vi "测试-图片插入word.vi"() -> ()   [LabVIEW 2018]
uses:
  <vilib>/Utility/NIReport.llb/Report Type.ctl
  <vilib>/Utility/NIReport.llb/Append Image to Report (path wrap).vi
  <vilib>/Utility/NIReport.llb/NI_report.lvclass
  <vilib>/Utility/NIReport.llb/Word/NI_Word.lvclass
  <vilib>/Utility/NIReport.llb/NI_ReportGenerationCore.lvlib
panel:
  out "报告生成路径 2":path
  out "报告生成路径":path
  out "标注图":T1(plugin-control)
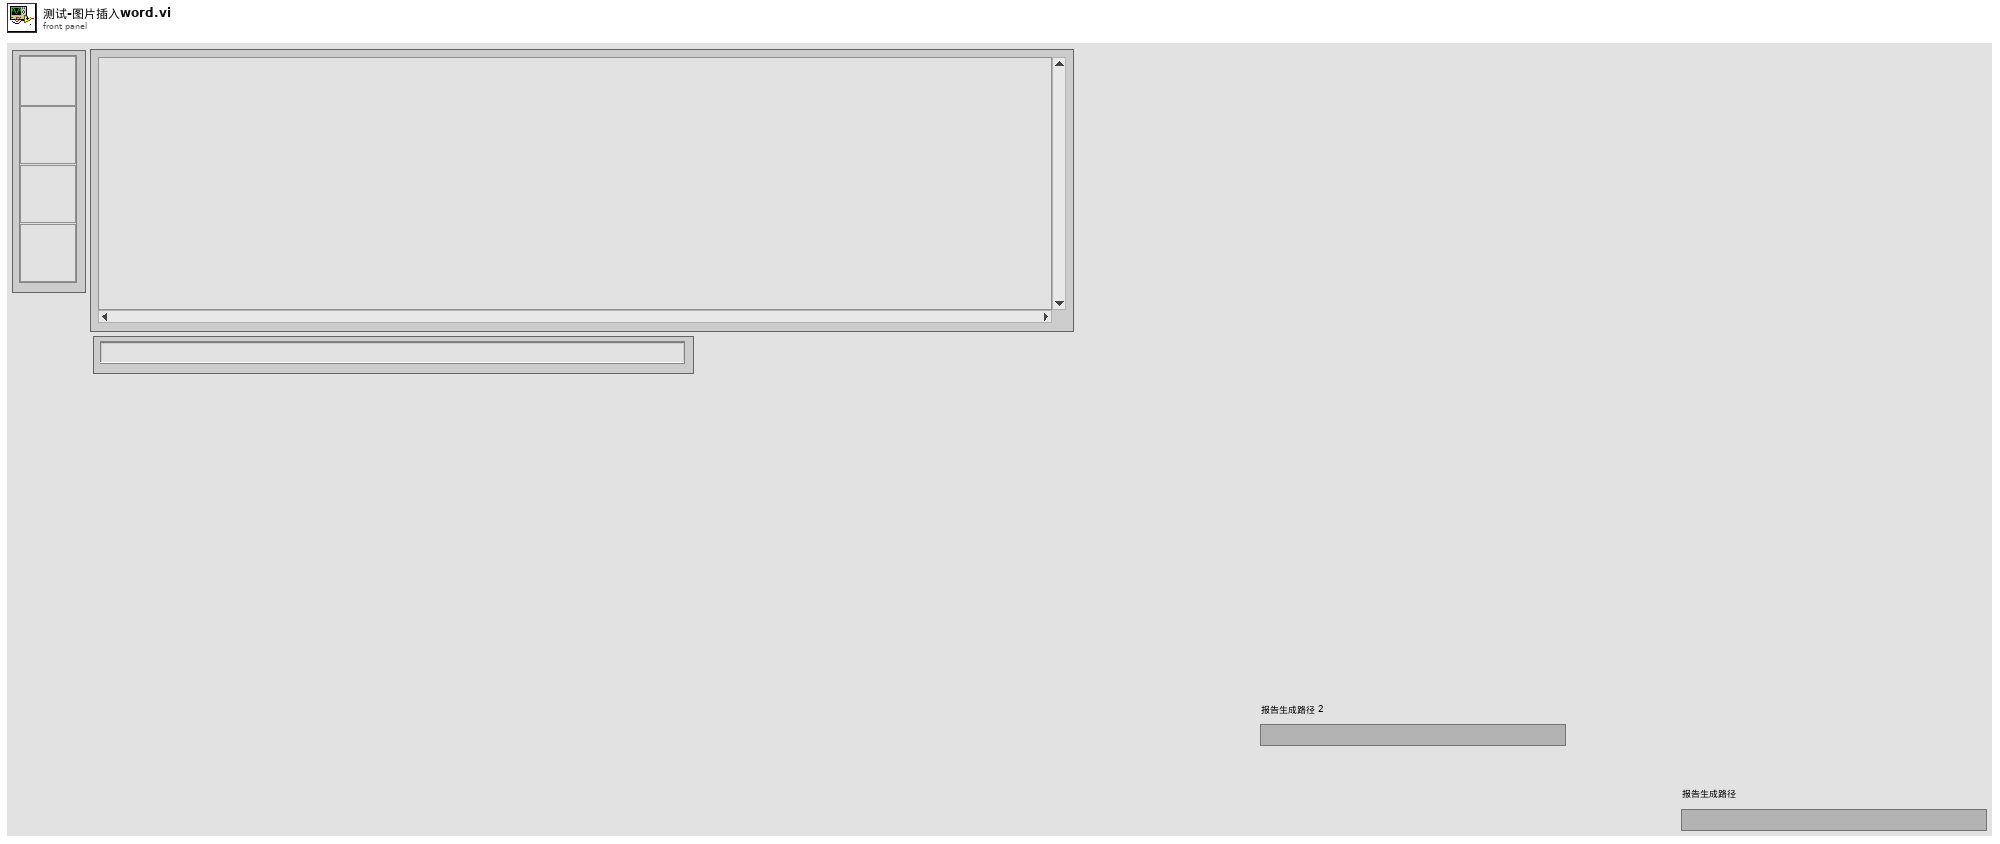
[diagram p1: front panel]
types:
  T1 = typedef "IMAQ Image.ctl" = refnum<image>
  T2 = cluster{"position (Excel)":cluster{"row":i32, "column":i32}, "name (Excel)":string, "bookmark (Word)":string}
  T3 = typedef "NI_ReportGenerationCore.lvlib/Report Type.ctl" = enum16{"HTML", "Word", "Excel"}
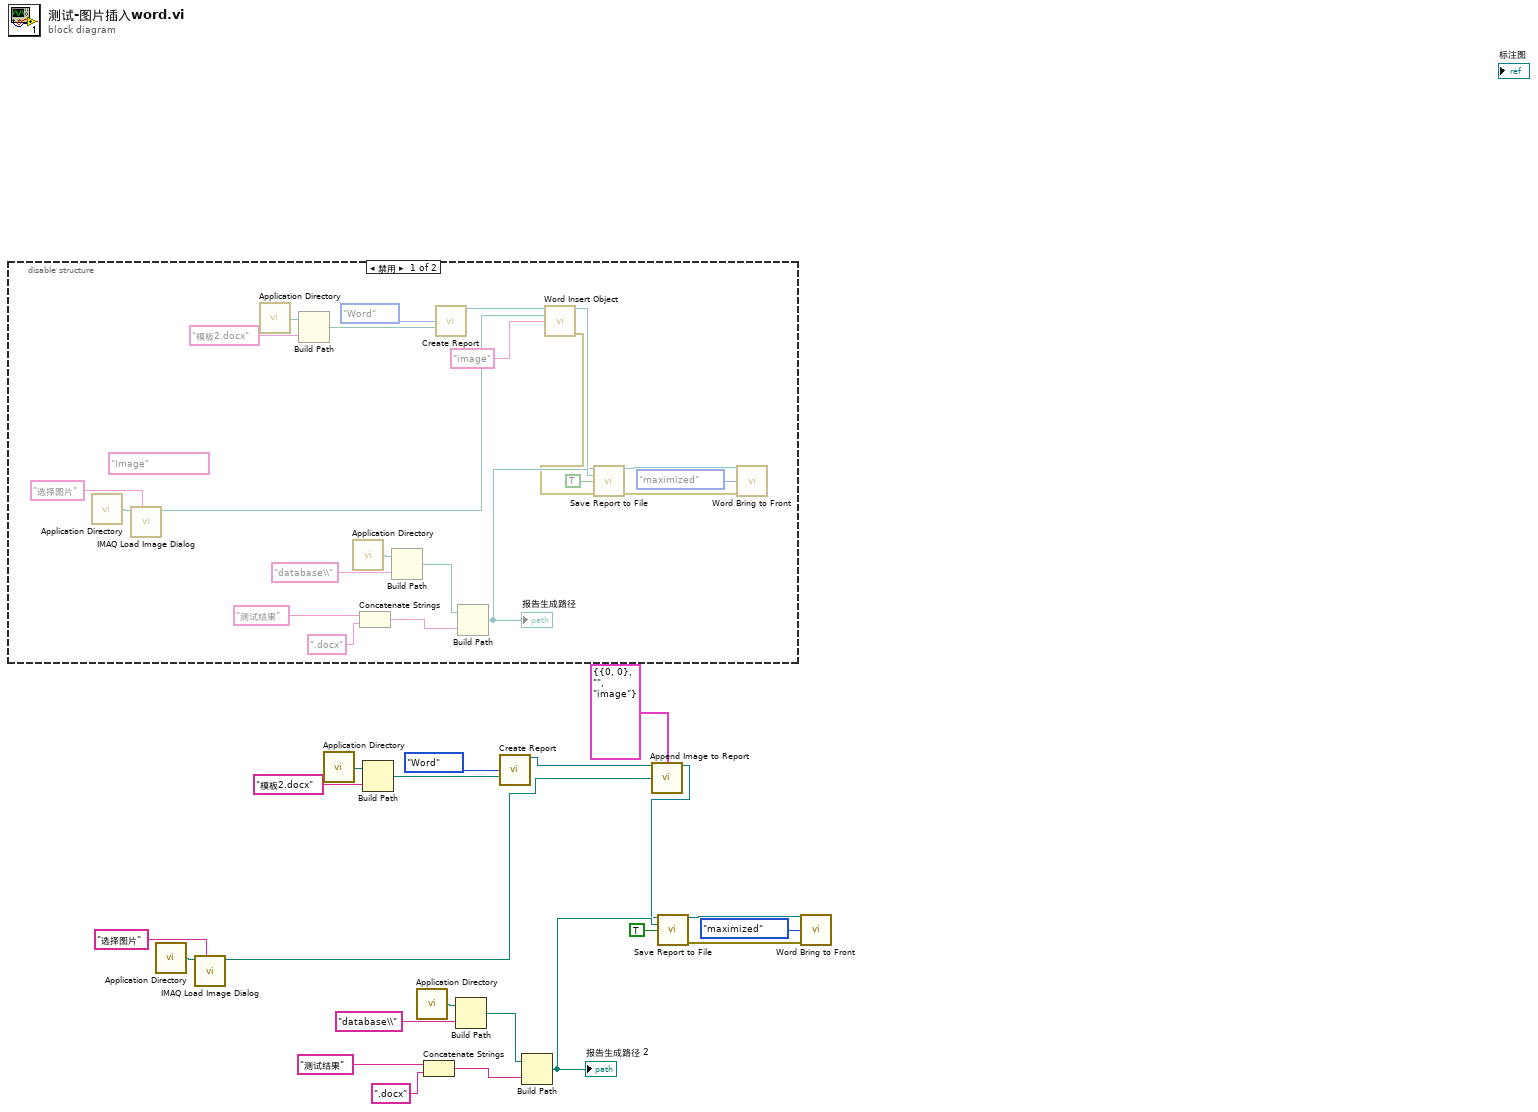
[diagram p0: block diagram]
diagram:
  n1 = disable-structure shown="禁用" {
    frame Disabled {
      (unwired) "Image" ("Image Name")
      n2 = call <vilib>:"Application Directory.vi"() -> ("Application Directory"=w38:path)
      n3 = call "IMAQ Load Image Dialog"("Prompt"="选择图片" ("prompt"), "Start Path"=w38) -> ("Path"=w36:path)  [unwired: 7 in, 2 out]
      n4 = call <vilib>:"Application Directory.vi"() -> ("Application Directory"=w43:path)
      n5 = Build Path(base path=w43, name or relative path="模板2.docx") -> (appended path=w42:path)
      n6 = call <vilib>:"Application Directory.vi"() -> ("Application Directory"=w32:path)
      n7 = Concatenate Strings("测试结果" ("字符串"), ".docx" ("名称或相对路径")) -> (w34:string)
      n8 = Build Path(base path=w32, name or relative path="database\\" ("名称或相对路径")) -> (appended path=w25:path)
      n9 = call <vilib>:"Create Report.vi"("report type"=Report_Type."Word" ("Report Type"), "template (empty)"=w42) -> ("report out"=w39:refnum<class "NI_report.lvclass">)  [unwired: 12 in, 1 out]
      n10 = Build Path(base path=w25, name or relative path=w34) -> (appended path=w24:path)
      "报告生成路径" <- w24
      n11 = call <vilib>:"Word Insert Object.vi"("report in"=w39, "file path"=w36, "bookmark (\"\")"="image" ("bookmark (\"\")")) -> ("report out"=w23:refnum<class "NI_report.lvclass">, "error out"=w22:errorcluster)  [unwired: 11 in]
      n12 = call-dynamic "Save Report to File.vi"("report in"=w23, "report file path"=w24, "prompt to replace? (F)"=TRUE, "error in (no error)"=w22) -> ("report out"=w30:refnum<class "NI_report.lvclass">, "error out"=w29:errorcluster)  [unwired: 10 in]
      n13 = call <vilib>:"Word Bring to Front.vi"("report in"=w30, "window state (maximized)"=enum16{"maximized", "minimized", "normal"}."maximized", "error in (no error)"=w29) -> ()  [unwired: 11 in, 2 out]
    }
    frame Enabled {
    }
  }
  n14 = call <vilib>:"Application Directory.vi"() -> ("Application Directory"=w17:path)
  n15 = call "IMAQ Load Image Dialog"("Prompt"="选择图片" ("prompt"), "Start Path"=w17) -> ("Path"=w3:path)  [unwired: 7 in, 2 out]
  n16 = call <vilib>:"Application Directory.vi"() -> ("Application Directory"=w21:path)
  n17 = Build Path(base path=w21, name or relative path="模板2.docx") -> (appended path=w20:path)
  n18 = call <vilib>:"Application Directory.vi"() -> ("Application Directory"=w13:path)
  n19 = Concatenate Strings("测试结果" ("字符串"), ".docx" ("名称或相对路径")) -> (w15:string)
  n20 = Build Path(base path=w13, name or relative path="database\\" ("名称或相对路径")) -> (appended path=w6:path)
  n21 = call <vilib>:"Create Report.vi"("report type"=Report_Type."Word" ("Report Type"), "template (empty)"=w20) -> ("report out"=w4:refnum<class "NI_report.lvclass">)  [unwired: 12 in, 1 out]
  n22 = Build Path(base path=w6, name or relative path=w15) -> (appended path=w5:path)
  "报告生成路径 2" <- w5
  n23 = call-poly <vilib>:"Append Image to Report.vi"("report in"=w4, "MS Office parameters"=T2 {"position (Excel)"={"row"=0, "column"=0}, "name (Excel)"="", "bookmark (Word)"="image"}, "path or URL of image"=w3) -> ("report out"=w1:refnum<class "NI_report.lvclass">)  [unwired: 9 in, 3 out]
  n24 = call-dynamic "Save Report to File.vi"("report in"=w1, "report file path"=w5, "prompt to replace? (F)"=TRUE) -> ("report out"=w11:refnum<class "NI_report.lvclass">, "error out"=w10:errorcluster)  [unwired: 11 in]
  n25 = call <vilib>:"Word Bring to Front.vi"("report in"=w11, "window state (maximized)"=enum16{"maximized", "minimized", "normal"}."maximized", "error in (no error)"=w10) -> ()  [unwired: 11 in, 2 out]
